vi "CCDbasicShutterV0.1.vi"(3 "error in":errorcluster, 4 "Shutter Enabled":bool=TRUE, 5 "Exposure time":dbl=0.2 format="%.2f") -> (0 "error out":errorcluster, 1 "ExpTime string":string="ex0.20", 2 "ExpTime returned":dbl=0.2 format="%.2f")   [LabVIEW 2020]
doc: "Sets the exposure time and shutter action for the \nnext CCD shot. Exposure time is returned between \n0.02 and 6000s. This VI uses the Global variable \nCCDsetupGLOBAL.var for CCD GPIB address and \nexposure-time and -string as well as shutter action."
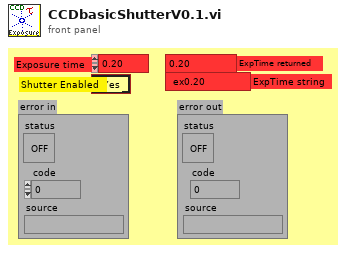
[diagram p1: front panel]
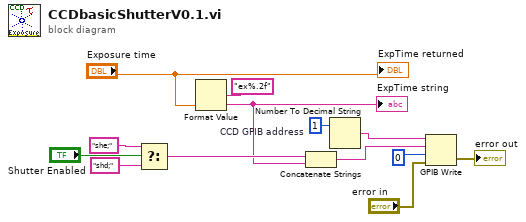
[diagram p0: block diagram]
diagram:
  w3 = 1  # CCD GPIB address
  n1 = Select(t="she;", s="Shutter Enabled", f="shd;") -> (s? t:f=w12:string)
  n2 = Format Value(format string="ex%.2f", value (0)="Exposure time") -> (output string=w8:string)  [unwired: 1 in]
  "ExpTime string" <- w8
  n3 = Concatenate Strings(w12, w8) -> (w6:string)
  n4 = Number To Decimal String(number=w3) -> (decimal integer string=w7:string)  [unwired: 1 in]
  n5 = GPIB Write(0:w7, 1:w6, 2:u8 0, 3:"error in") -> (6:→"error out":errorcluster)  [unwired: 1 in, 1 out]
  "ExpTime returned" <- "Exposure time"
